vi "DrawGsphere.vi"(0 "Object in":refnum<vi>, 2 "contents":string, 3 "Color":T1={"Red"=0.0, "Green"=0.0, "Blue"=1.0, "Alpha"=1.0}) -> (1 "Object out":refnum<vi>, 4 "remaining":string)   [LabVIEW 2012]
uses:
  <vilib>/picture/3D Picture Control/NI_3D Picture Control.lvlib
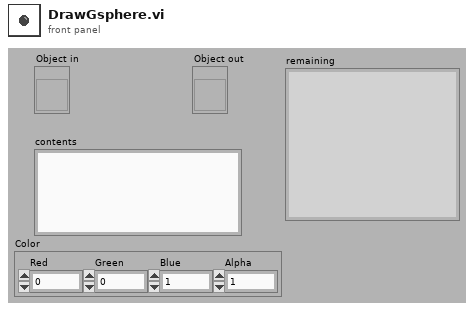
[diagram p1: front panel]
types:
  T1 = cluster{"Red":sgl, "Green":sgl, "Blue":sgl, "Alpha":sgl}
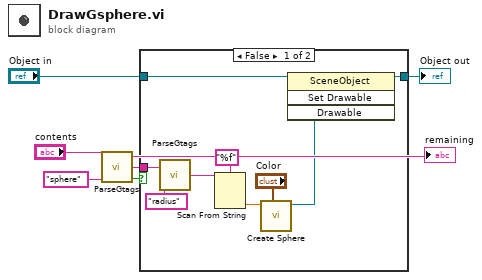
[diagram p0: block diagram]
diagram:
  n1 = call <userlib>:"ParseGtags.vi"("tag"="sphere", "urdf in"="contents") -> ("not found"=w4:bool, "contents"=w5:string, "urdf out"=→"remaining":string)  [unwired: 1 out]
  n2 = case shown="False" w4 {
    tunnel: w5 -> [w15 _]
    tunnel: "Object in" -> [w13 w17]
    tunnel: [w12 w17] -> w7
    frame False {
      n3 = call <userlib>:"ParseGtags.vi"("tag"="radius", "urdf in"=w15) -> ("contents"=w14:string)  [unwired: 3 out]
      n4 = Scan From String(format string="%f", input string=w14) -> (output 1=w9:dbl)  [unwired: 3 in, 3 out]
      n5 = call <vilib>:"Create Sphere.vi"("Color"="Color", "Radius"=w9) -> ("New Sphere Refnum"=w10:refnum<vi>)  [unwired: 8 in, 1 out]
      n6 = invoke class="SceneObject" method="Set Drawable"(reference=w13, "Drawable"=w10) -> (reference out=w12:refnum<vi>)  [unwired: 2 in, 3 out]
    }
    frame True {
    }
  }
  "Object out" <- w7
